vi "test- async-resp for csm loop.vi"(8 "error in (no error)":errorcluster, 11 "TestCase in":refnum<class "testcase-csm loop support.lvclass">) -> (0 "error out":errorcluster, 3 "TestCase out":refnum<class "testcase-csm loop support.lvclass">)   [LabVIEW 2017, in "testcase-csm loop support.lvclass"]
uses:
  testcase-csm loop support.lvclass
  56d4bdba-c2f1-4b55-add1-7a078de9da03.vi
  ea54eaf7-6c78-4206-8259-080cdfbb85de.vi
  src/user.lib/_NEVSTOP/Communicable State Machine(CSM)/AdvanceAPI/CSM - Revert Arguments-Safe String.vi
  src/user.lib/_NEVSTOP/Communicable State Machine(CSM)/_Shared/Trim Single-line Text.vi
  src/user.lib/_NEVSTOP/Communicable State Machine(CSM)/AdvanceAPI/CSM - Make String Arguments Safe.vi
  src/user.lib/_NEVSTOP/Communicable State Machine(CSM)/AdvanceAPI/CSM - Break Down Multiple States String.vi
  src/user.lib/_NEVSTOP/Communicable State Machine(CSM)/AdvanceAPI/CSM - Compact Multiple States.vi
  src/user.lib/_NEVSTOP/Communicable State Machine(CSM)/AdvanceAPI/CSM - Keywords.vi
  <vilib>/addons/_JKI Toolkits/VI Tester/TestCase.llb/TestCase.lvclass
  src/user.lib/_NEVSTOP/Communicable State Machine(CSM)/Communicable State Machine.lvlib
  src/user.lib/_NEVSTOP/Communicable State Machine(CSM)/addons/Loop-Support/CSM Loop Support.lvlib
  C:/Program Files (x86)/National Instruments/LabVIEW 2017/vi.lib/addons/_JKI Toolkits/VI Tester/TestCase.llb/TestCase.lvclass
panel:
  out "Arguments":string
  out "State History 2":string
  out "State History":string
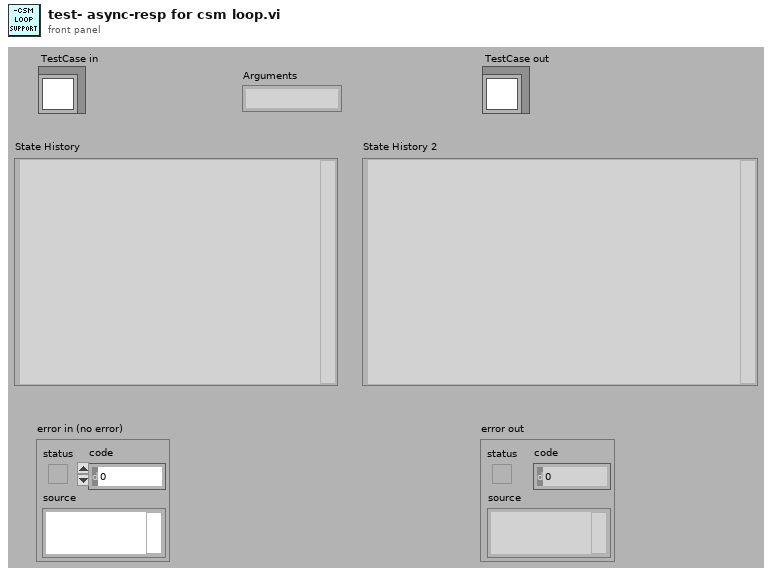
[diagram p1: front panel]
types:
  T1 = enum32{"Invalid", "Standard", "Closed", "Hidden", "Minimized", "Maximized"}
  T2 = enum32{"invalid app kind", "Development System", "Run Time System", "Student Edition", "Embedded LabVIEW", "Evaluation", "Custom"}
  T3 = typedef "Communicable State Machine.lvlib/_CSM_Response Source Message.ctl" = cluster{"‘State":string, "’Arguments":string, "’Error":errorcluster}
  T4 = cluster{"Current VI Reference":refnum<vi>, "Close Panel on Exit?":bool}
  T5 = cluster{"Core":cluster{"Current VI Reference":refnum<vi>, "Close Panel on Exit?":bool}, "diff":dbl, "time":timestamp}
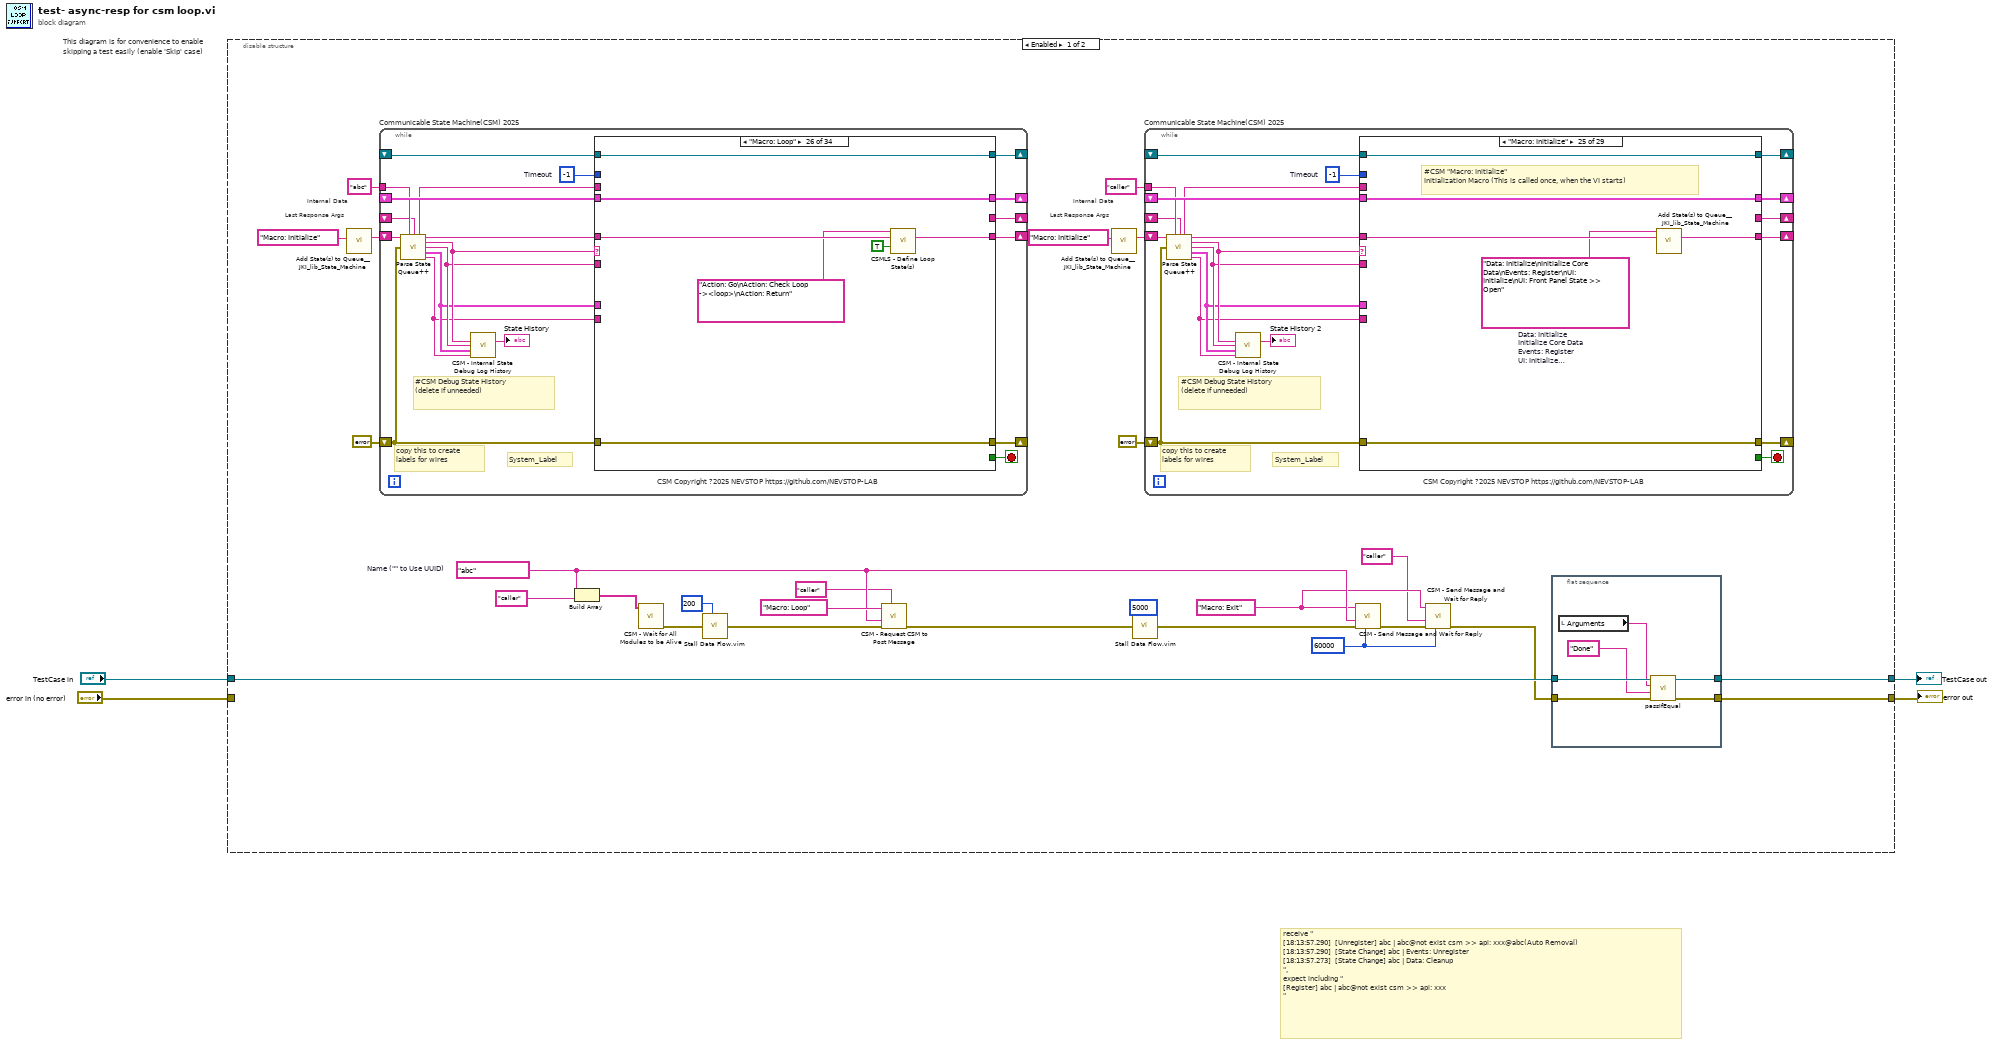
[diagram p0: block diagram]
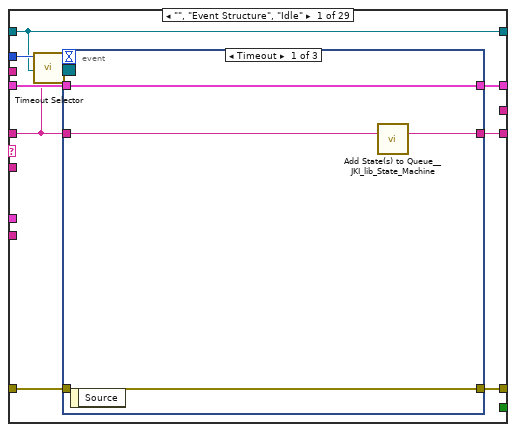
[diagram p2: hidden frame]
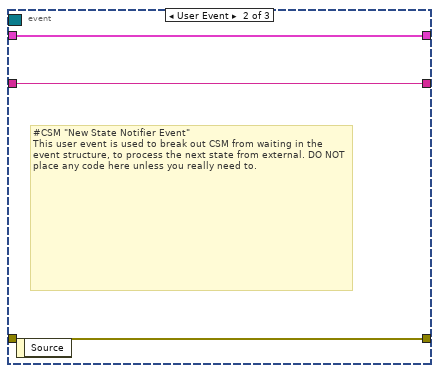
[diagram p3: hidden frame]
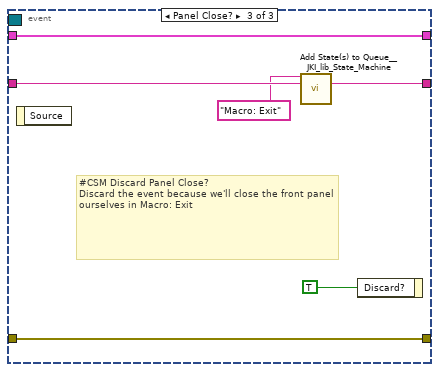
[diagram p4: hidden frame]
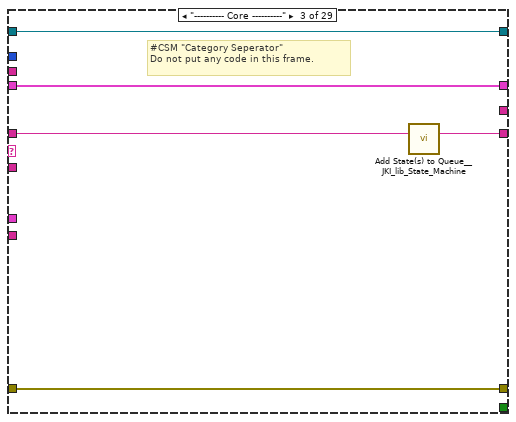
[diagram p6: hidden frame]
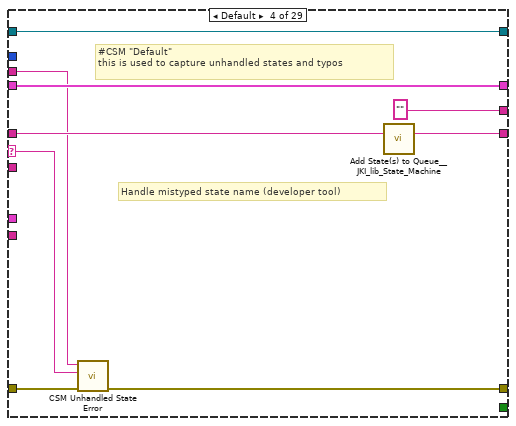
[diagram p7: hidden frame]
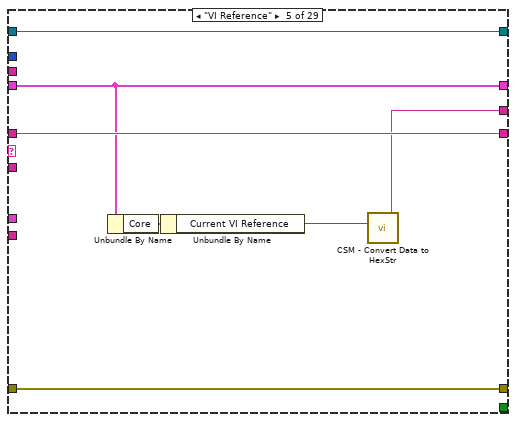
[diagram p8: hidden frame]
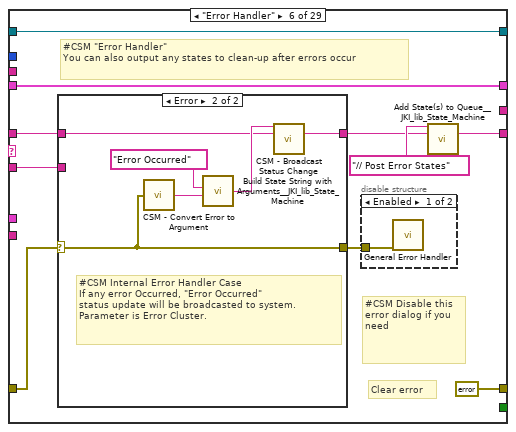
[diagram p9: hidden frame]
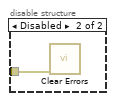
[diagram p10: hidden frame]
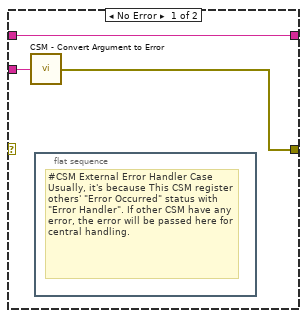
[diagram p11: hidden frame]
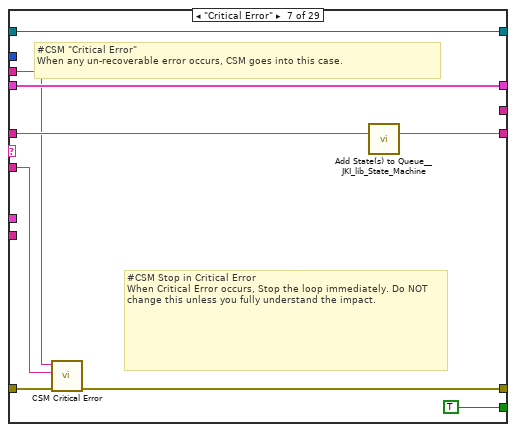
[diagram p12: hidden frame]
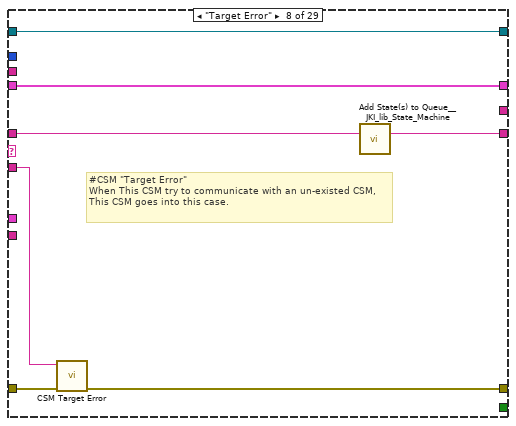
[diagram p13: hidden frame]
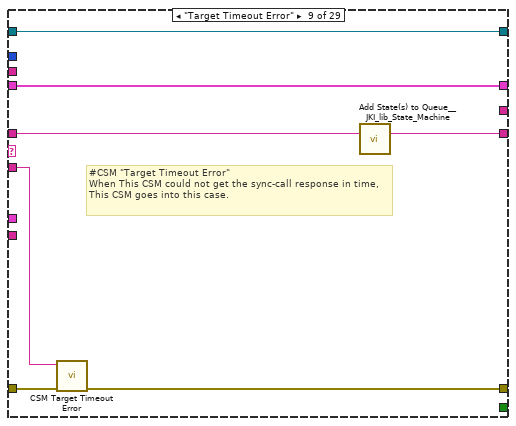
[diagram p14: hidden frame]
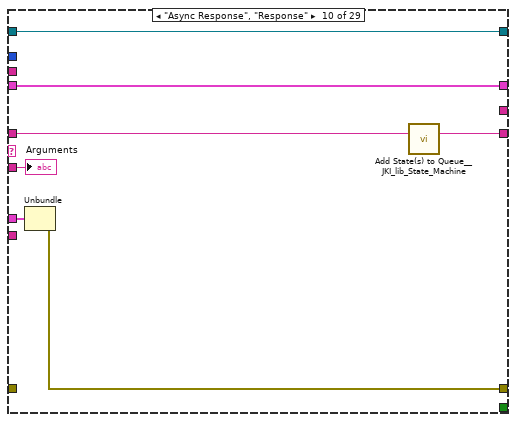
[diagram p15: hidden frame]
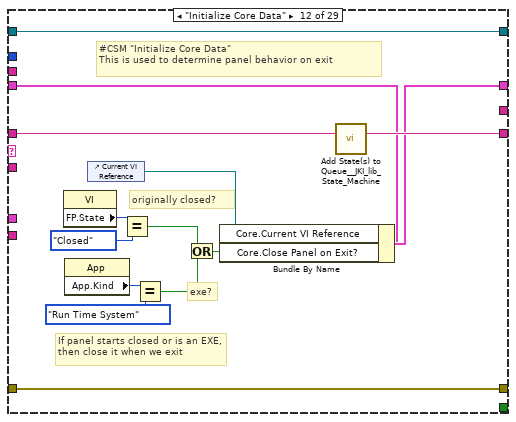
[diagram p17: hidden frame]
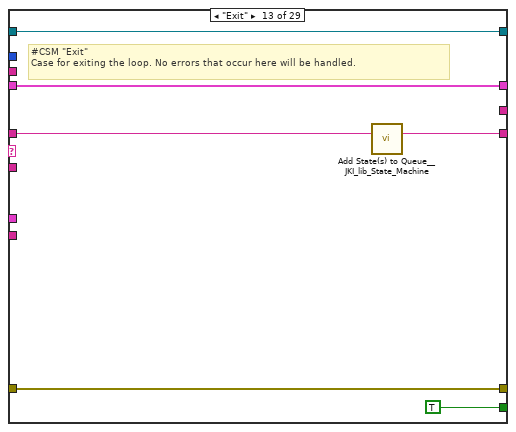
[diagram p18: hidden frame]
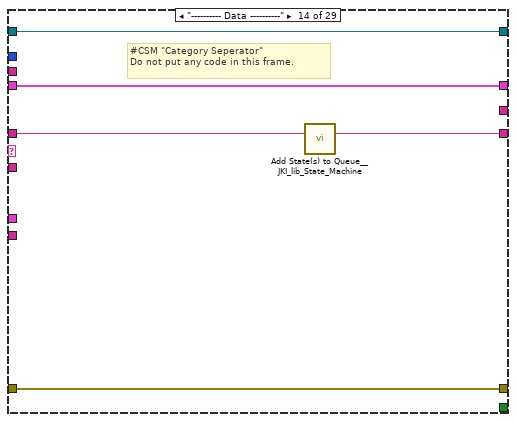
[diagram p19: hidden frame]
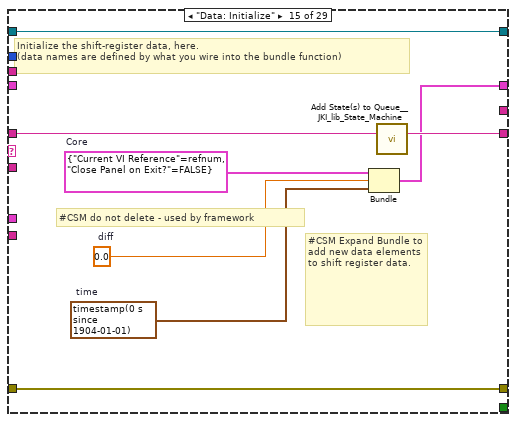
[diagram p20: hidden frame]
diagram:
  # "receive \"\n[18:13:57.290]  [Unregister] abc | abc@not exist csm >> api: xxx@abc(Auto Removal)\n[18:13:57.290]  [State Change] abc | Events: Unregister\n[18:13:57.273]  [State Change] abc | Data: Cleanup\n\", \nexpect including \"\n[Register] abc | abc@not exist csm >> api: xxx\n\""
  n1 = disable-structure "This diagram is for convenience to enable skipping a test easily (enable 'Skip' case)" shown="Enabled" {
    disable-tunnel: "TestCase in" -> [w24 w727]
    disable-tunnel: [w23 w725] -> w1
    disable-tunnel: [w22 w726] -> w3
    disable-tunnel: "error in (no error)" -> [_ w724]
    frame Enabled {
      w5 = 60000 ("Response Timeout (-2 Using Global Settings)")
      w8 = "Macro: Exit" ("State")
      w11 = "abc"  # Name ("" to Use UUID)
      # "Last Response Args"
      # "Internal Data"
      # "Last Response Args"
      # "Internal Data"
      n2 = call <vilib>:"Add State(s) to Queue__JKI_lib_State_Machine.vi"("State(s) in (\"\")"="Macro: Initialize" ("Init State(\"Macro: Initialize\")")) -> ("States Out"=w30:string)  [unwired: 14 in]
      n3 = while "Communicable State Machine(CSM) 2025" {
        shift-right: [w370] -> _
        shift-left: _ -> [w369]
        shift-right: [w373] -> _
        shift-left: errorcluster {"status"=FALSE, "code"=0, "source"=""} ("error out") -> [w367]
        shift-right: [w372] -> _
        shift-left: w30 -> [w374]
        tunnel: "abc" ("Name (\"\" to Use UUID)") -> [w363]
        shift-right: [w366] -> _
        shift-left: _ -> [w357]
        shift-right: [w365] -> _
        shift-left: _ -> [w364]
        stop <- w371 stop-if-true
        w368 = -1  # Timeout
        # "#CSM Debug State History\n(delete if unneeded)"
        # "copy this to create labels for wires"
        # "System_Label"
        # "CSM Copyright ?2025 NEVSTOP https://github.com/NEVSTOP-LAB"
        n4 = call "Parse State Queue++.vi"("State Queue"=w374, "Name (\"\" to Use UUID)"=w363, "Response Arguments"=w357, "Previous Error"=w367) -> ("Name Used"=w358:string, "Remaining States"=w375:string, "Current State"=w362:string, "Arguments"=w361:string, "Additional Information"=w360:T3, "Source CSM"=w359:string)  [unwired: 6 in]
        n5 = call "CSM - Internal State Debug Log History.vi"("State"=w362, "Arguments (\"\")"=w361, ">> Response Source Message >>"=w360, "Source (\"\")"=w359) -> ("Debug Log"=→"State History":string)  [unwired: 11 in]
        n6 = case shown="\"Macro: Loop\"" w362 {
          selector: w362 -> [_ _ _ w409 _ _ _ _ _ _ _ _ _ _ _ _ _ _ _ _ _ _ _ _ _ _ _ _ _ _ _ _ w709 _]
          tunnel: w375 -> [w376 w400 w406 w414 w421 w427 w450 w456 w463 w472 w485 w500 w506 w511 w519 w526 w531 w538 w542 w548 w553 w560 w576 w646 w652 w659 w671 w674 w679 w685 w693 w700 w710 w722]
          tunnel: w361 -> [_ _ _ _ _ w426 w445 w455 w462 w471 _ _ _ _ _ _ _ _ _ _ _ w555 w570 _ _ _ _ _ _ w682 _ _ _ _]
          tunnel: w369 -> [w383 w399 w403 w412 w420 w431 w451 w458 w465 w474 w484 w493 w504 w508 _ w521 w528 w537 w541 w545 w551 w558 w572 w643 w649 w656 w668 w673 w678 w684 w690 w697 w706 w720]
          tunnel: [w382 w401 w404 w407 w422 errorcluster {"status"=FALSE, "code"=0, "source"=""} ("error out") w446 w453 w460 w477 w486 w497 w503 w509 w516 w522 w529 w532 w540 w546 w550 w556 w573 w644 w650 w657 w669 w675 w680 w686 w691 w698 w712 w723] -> w373
          tunnel: w367 -> [w381 w401 w404 w415 w422 w428 w452 w454 w461 _ w486 w497 w503 w509 w516 w523 w529 _ w543 w546 w550 w557 w574 w644 w650 w657 w669 w675 w680 w686 w691 w698 w712 w723]
          tunnel: [w384 w400 w405 w413 w421 w423 w449 w459 w466 w473 w485 w499 w505 w510 w518 w525 w530 w538 w542 w547 w552 w559 w575 w645 w651 w658 w670 w674 w679 w685 w692 w699 w713 w722] -> w372
          tunnel: [_ _ _ _ _ _ TRUE _ _ _ _ _ TRUE _ _ _ _ _ _ _ _ _ _ _ _ _ _ _ _ _ _ _ _ _] -> w371
          tunnel: [w380 w399 w403 w412 w420 w431 w451 w458 w465 w475 w484 w498 w504 w508 w517 w521 w528 w537 w541 w545 w551 w558 w572 w643 w649 w656 w668 w673 w678 w684 w690 w695 w702 w720] -> w370
          tunnel: w368 -> [w379 _ _ _ _ _ _ _ _ _ _ _ _ _ _ _ _ _ _ _ _ _ _ _ _ _ _ _ _ _ _ _ _ _]
          tunnel: w359 -> [_ _ _ _ _ _ _ _ _ w469 _ _ _ _ _ _ _ _ _ _ _ _ _ _ _ _ _ _ _ _ _ _ _ _]
          tunnel: w360 -> [_ _ _ _ _ _ _ _ _ w476 _ _ _ _ _ _ _ _ _ _ _ _ _ _ _ _ _ _ _ _ _ _ _ _]
          tunnel: [_ _ _ "" w416 _ _ _ _ _ _ _ _ _ _ _ _ _ _ _ _ _ _ _ _ _ _ _ "API1 Response" w681 _ _ _ "Done" ("HEX String (0-9,A-F)")] -> w366
          tunnel: [w378 w398 w402 w410 w419 w430 w447 w457 w464 w478 w483 w487 w501 w507 w512 w520 w527 w536 w539 w544 w549 w554 w569 w642 w647 w654 w661 w672 w677 w683 w689 w696 w711 w721] -> w365
          tunnel: w364 -> [w378 w398 w402 w410 w419 w430 w447 w457 w464 w478 w483 w487 w501 w507 w512 w520 w527 _ w539 w544 w549 w554 w569 w642 w647 w654 w661 w672 w677 w683 w689 w696 w711 w721]
          tunnel: w358 -> [_ _ _ w408 _ _ w444 _ _ _ _ _ _ _ _ _ _ w535 _ _ _ _ _ _ _ _ _ _ _ _ _ _ _ _]
          frame "", "Event Structure", "Idle" {
            n7 = call "Timeout Selector.vi"("Remaining States"=w376, "Timeout Expected"=w379) -> ("Timeout"=w377:i32)  [unwired: 5 in]
            n8 = event shown="[1] <New State Notifier Event>: User Event" {
              selector: w378 -> [_ _ _]
              dyn-events: _ -> [_ _ _]
              timeout: w377 -> [_ _ _]
              tunnel: w376 -> [w388 w390 w397]
              tunnel: [w387 w390 w396] -> w384
              tunnel: w383 -> [w385 w391 w394]
              tunnel: [w386 w389 w395] -> w382
              tunnel: w381 -> [w386 w389 w395]
              tunnel: [w385 w391 w394] -> w380
              event Timeout {
                n9 = event-data() -> ()  [unwired: 1 in, 1 out]
                n10 = call <vilib>:"Add State(s) to Queue__JKI_lib_State_Machine.vi"("State(s) in (\"\")"=w388) -> ("States Out"=w387:string)  [unwired: 14 in]
              }
              event User Event {
                # "#CSM \"New State Notifier Event\"\nThis user event is used to break out CSM from waiting in the event structure, to process the next state from external. DO NOT place any code here unless you really need to."
                n11 = event-data() -> ()  [unwired: 1 in, 1 out]
              }
              event Panel Close? {
                # "#CSM Discard Panel Close?\nDiscard the event because we'll close the front panel ourselves in Macro: Exit"
                n12 = event-data() -> ()  [unwired: 1 in, 1 out]
                n13 = call <vilib>:"Add State(s) to Queue__JKI_lib_State_Machine.vi"("State(s) in Front (\"\")"="Macro: Exit", "State(s) in (\"\")"=w397) -> ("States Out"=w396:string)  [unwired: 13 in]
                n14 = event-data("Discard?"=TRUE) -> ()  [unwired: 1 in, 1 out]
              }
            }
          }
          frame "CSM Documentation" {
            # "#CSM README FIRST\n\nCommunicable State Machine(CSM) is a LabVIEW application framework that builds upon JKI State Machine(JKISM). It follows the pattern of JKISM and extends the keywords to describe message communication between modules, including concepts such as Sync-Message, Async-Message, Subscription/Unsubscription of status - essential elements for creating reusable code modules. For more information, please visit the CSM wiki: https://nevstop-lab.github.io/CSM-Wiki/\n\nFor instructions on JKI State Machine, visit: http://jki.net/state-machine/\nFor information about CSM, visit: https://github.com/NEVSTOP-LAB"
            # "#CSM \"Documentation\"\nCase for holding CSM Documenation"
          }
          frame "---------- Core ----------" {
            # "#CSM \"Category Seperator\"\nDo not put any code in this frame."
            n15 = call <vilib>:"Add State(s) to Queue__JKI_lib_State_Machine.vi"("State(s) in (\"\")"=w406) -> ("States Out"=w405:string)  [unwired: 14 in]
          }
          frame Default {
            # "#CSM \"Default\"\nthis is used to capture unhandled states and typos"
            # "Handle mistyped state name (developer tool)"
            n16 = call "CSM Unhandled State Error.vi"("error in (no error)"=w415, "Undefined State"=w409, "CSM Name"=w408) -> ("error out"=w407:errorcluster)  [unwired: 8 in]
            n17 = call <vilib>:"Add State(s) to Queue__JKI_lib_State_Machine.vi"("State(s) in (\"\")"=w414) -> ("States Out"=w413:string)  [unwired: 14 in]
          }
          frame "VI Reference" {
            n18 = Unbundle By Name(w420) -> ("Core"=w418:T4)
            n19 = Unbundle By Name(w418) -> ("Current VI Reference"=w417:refnum<vi>)
            n20 = call "CSM - Convert Data to HexStr.vi"("Variant"=w417) -> ("HEX String (0-9,A-F)"=w416:string)  [unwired: 8 in]
          }
          frame "Error Handler" {
            # "#CSM Disable this error dialog if you need"
            # "#CSM \"Error Handler\"\nYou can also output any states to clean-up after errors occur"
            # "Clear error"
            n21 = case shown="Error" w428 {
              selector: w428 -> [_ w438]
              tunnel: [w437 w440] -> w424
              tunnel: w427 -> [w437 w439]
              tunnel: w426 -> [w436 _]
              tunnel: [w435 w438] -> w429
              frame No Error {
                n22 = call "CSM - Convert Argument to Error.vi"("Argument"=w436) -> ("Error"=w435:errorcluster)  [unwired: 4 in]
                n23 = flat-sequence {
                  frame #0 {
                    # "#CSM External Error Handler Case\nUsually, it's because This CSM register others' \"Error Occurred\" status with \"Error Handler\". If other CSM have any error, the error will be passed here for central handling."
                  }
                }
              }
              frame Error {
                # "#CSM Internal Error Handler Case \nIf any error Occurred, \"Error Occurred\" \nstatus update will be broadcasted to system.\nParameter is Error Cluster."
                n24 = call "CSM - Convert Error to Argument.vi"("Error"=w438) -> ("Argument"=w442:string)  [unwired: 4 in]
                n25 = call <vilib>:"Build State String with Arguments__JKI_lib_State_Machine.vi"("Arguments (\"\")"=w442, "State"="Error Occurred" ("Status with Arguments")) -> ("State with Arguments"=w441:string)  [unwired: 4 in]
                n26 = call "CSM - Broadcast Status Change.vi"("Status With Arguments"=w441, "State Queue"=w439) -> ("Remaining States"=w440:string)  [unwired: 13 in]
              }
            }
            n27 = disable-structure shown="Enabled" {
              disable-tunnel: w429 -> [w433 w434]
              frame Enabled {
                n28 = call <vilib>:"General Error Handler.vi"("error in (no error)"=w433) -> ()  [unwired: 10 in, 5 out]
              }
              frame Disabled {
                n29 = call <vilib>:"Clear Errors.vi"("error in (no error)"=w434) -> ()  [unwired: 5 in, 2 out]
              }
            }
            n30 = call <vilib>:"Add State(s) to Queue__JKI_lib_State_Machine.vi"("State(s) in Front (\"\")"="// Post Error States", "State(s) in (\"\")"=w424) -> ("States Out"=w423:string)  [unwired: 13 in]
          }
          frame "Critical Error" {
            # "#CSM Stop in Critical Error\nWhen Critical Error occurs, Stop the loop immediately. Do NOT change this unless you fully understand the impact."
            # "#CSM \"Critical Error\"\nWhen any un-recoverable error occurs, CSM goes into this case."
            n31 = call "CSM Critical Error.vi"("error in (no error)"=w452, "Arugments (As Reason)"=w445, "CSM Name"=w444) -> ("error out"=w446:errorcluster)  [unwired: 8 in]
            n32 = call <vilib>:"Add State(s) to Queue__JKI_lib_State_Machine.vi"("State(s) in (\"\")"=w450) -> ("States Out"=w449:string)  [unwired: 14 in]
          }
          frame "Target Error" {
            # "#CSM \"Target Error\"\nWhen This CSM try to communicate with an un-existed CSM, This CSM goes into this case."
            n33 = call "CSM Target Error.vi"("error in (no error)"=w454, "Arguments (As CSM Name)"=w455) -> ("error out"=w453:errorcluster)  [unwired: 9 in]
            n34 = call <vilib>:"Add State(s) to Queue__JKI_lib_State_Machine.vi"("State(s) in (\"\")"=w456) -> ("States Out"=w459:string)  [unwired: 14 in]
          }
          frame "Target Timeout Error" {
            # "#CSM \"Target Timeout Error\"\nWhen This CSM could not get the sync-call response in time, This CSM goes into this case."
            n35 = call "CSM Target Timeout Error.vi"("error in (no error)"=w461, "Arguments (As CSM Name)"=w462) -> ("error out"=w460:errorcluster)  [unwired: 9 in]
            n36 = call <vilib>:"Add State(s) to Queue__JKI_lib_State_Machine.vi"("State(s) in (\"\")"=w463) -> ("States Out"=w466:string)  [unwired: 14 in]
          }
          frame "Async Response", "Response" {
            n37 = Unbundle(w476) -> ("‘State"=w470:string, "’Arguments"=w468:string, "’Error"=w467:errorcluster)
            n38 = case shown="Default" w470 {
              tunnel: [w482] -> w477
              tunnel: w467 -> [w482]
              tunnel: [w481] -> w475
              tunnel: w474 -> [w481]
              tunnel: [w479] -> w473
              tunnel: w472 -> [w480]
              tunnel: w471 -> [_]
              tunnel: w469 -> [_]
              tunnel: w468 -> [_]
              frame Default {
                # "#CSM Response Comments\nAfter Message is executed, CSM goes to this state for receive the response.\n    For Async Message(->), \"Async Response\" is used. This CSM will goes to \"Async Message Posted\" immediately and receive the \"Async Response\" after the callee finishes the message.\n    For Sync Message(@),  This CSM will wait until the message is done and immediately goes to \"Response\""
                # "#CSM \"Async Response\"\nHandle Async-call Response (\"Async Response\" for ->)"
                # "#CSM \"Response\"\nHandle Sync-call Response (\"Response\" for -@)"
                n39 = call <vilib>:"Add State(s) to Queue__JKI_lib_State_Machine.vi"("State(s) in (\"\")"=w480) -> ("States Out"=w479:string)  [unwired: 14 in]
              }
            }
          }
          frame "Async Message Posted" {
            # "#CSM \"Async Message Posted\"\nAfter Async Message is posted (-> or ->| ), CSM goes to this state for post-action.\nYou can use Argument - State to tell which Async Message is called."
          }
          frame "Initialize Core Data" {
            # "#CSM \"Initialize Core Data\"\nThis is used to determine panel behavior on exit"
            # "originally closed?"
            # "exe?"
            # "If panel starts closed or is an EXE, then close it when we exit"
            n40 = property class="VI"() -> ("FP.State"=w490:T1)  [unwired: 2 in, 2 out]
            n41 = property class="App"() -> ("App.Kind"=w496:T2)  [unwired: 2 in, 2 out]
            n42 = control-ref of="Current VI Reference"() -> (w491:refnum<vi>)
            n43 = Equal?(x=w490, y=T1."Closed" ("Front Panel Window:State")) -> (x = y?=w488:bool)
            n44 = Equal?(x=w496, y=T2."Run Time System" ("Application:Kind")) -> (x = y?=w494:bool)
            n45 = Or(x=w488, y=w494) -> (x .or. y?=w492:bool)
            n46 = Bundle By Name(cluster=w493, "Core.Current VI Reference"=w491, "Core.Close Panel on Exit?"=w492) -> (w498:T5)
            n47 = call <vilib>:"Add State(s) to Queue__JKI_lib_State_Machine.vi"("State(s) in (\"\")"=w500) -> ("States Out"=w499:string)  [unwired: 14 in]
          }
          frame "Exit" {
            # "#CSM \"Exit\"\nCase for exiting the loop. No errors that occur here will be handled."
            n48 = call <vilib>:"Add State(s) to Queue__JKI_lib_State_Machine.vi"("State(s) in (\"\")"=w506) -> ("States Out"=w505:string)  [unwired: 14 in]
          }
          frame "---------- Data ----------" {
            # "#CSM \"Category Seperator\"\nDo not put any code in this frame."
            n49 = call <vilib>:"Add State(s) to Queue__JKI_lib_State_Machine.vi"("State(s) in (\"\")"=w511) -> ("States Out"=w510:string)  [unwired: 14 in]
          }
          frame "Data: Initialize" {
            w513 = T4 {"Current VI Reference"=refnum, "Close Panel on Exit?"=FALSE}  # Core
            w515 = 0.0  # diff
            w514 = timestamp(0 s since 1904-01-01)  # time
            # "#CSM do not delete - used by framework"
            # "#CSM Expand Bundle to add new data elements to shift register data."
            # "Initialize the shift-register data, here.\n(data names are defined by what you wire into the bundle function)"
            n50 = Bundle("Core"=w513, "diff"=w515, "time"=w514) -> (w517:T5)  [unwired: 1 in]
            n51 = call <vilib>:"Add State(s) to Queue__JKI_lib_State_Machine.vi"("State(s) in (\"\")"=w519) -> ("States Out"=w518:string)  [unwired: 14 in]
          }
          frame "Data: Cleanup" {
            # "Cleanup any data and references, here.\n(this is called automatically, by the Macro: Exit)"
            n52 = Unbundle By Name(w521) -> ("Core.Current VI Reference"=w524:refnum<vi>)
            n53 = Close Reference(reference=w524, error in (no error)=w523) -> (error out=w522:errorcluster)
            n54 = call <vilib>:"Add State(s) to Queue__JKI_lib_State_Machine.vi"("State(s) in (\"\")"=w526) -> ("States Out"=w525:string)  [unwired: 14 in]
          }
          frame "---------- Events ----------" {
            # "#CSM \"Category Seperator\"\nDo not put any code in this frame."
            n55 = call <vilib>:"Add State(s) to Queue__JKI_lib_State_Machine.vi"("State(s) in (\"\")"=w531) -> ("States Out"=w530:string)  [unwired: 14 in]
          }
          frame "Events: Register" {
            # "#CSM \"Events: Register\"\nRegister user event. New Message Event is registered to break CSM waiting in event structure by default."
            # "#CSM Register New Message Event\nRegister message event to break Waiting in Event structure."
            n56 = call "CSM - Get New State Notifier Event.vi"("Name (\"\" to Use UUID)"=w535) -> ("error out"=w533:errorcluster, "New State Notifier Event"=w534:refnum<user-event>)  [unwired: 9 in]
            n57 = register-events(error in=w533, w534) -> (reference out=w536:refnum<event-registration>, error out=w532:errorcluster)  [unwired: 1 in]
          }
          frame "Events: Unregister" {
            # "#CSM \"Events: Unregister\"\nUnregister user event."
            n58 = Unregister For Events(event registration refnum=w539, error in=w543) -> (error out=w540:errorcluster)
          }
          frame "---------- UI ----------" {
            # "#CSM \"Category Seperator\"\nDo not put any code in this frame."
            n59 = call <vilib>:"Add State(s) to Queue__JKI_lib_State_Machine.vi"("State(s) in (\"\")"=w548) -> ("States Out"=w547:string)  [unwired: 14 in]
          }
          frame "UI: Initialize" {
            # "#CSM \"UI: Initialize\"\nInitialize the User Interface, here.\n(this is called automatically, by the Macro: Init)"
            n60 = call <vilib>:"Add State(s) to Queue__JKI_lib_State_Machine.vi"("State(s) in (\"\")"=w553) -> ("States Out"=w552:string)  [unwired: 14 in]
          }
          frame "UI: Cursor Set" {
            # "#CSM \"UI: Cursor Set\"\nSet and Unset Cursor Busy.\n(Usage: \"UI: Cursor Set >> Busy|Idle\")"
            # "Argument"
            n61 = disable-structure shown="Default" {
              disable-tunnel: w557 -> [w563 w568]
              disable-tunnel: [w562 w568] -> w556
              disable-tunnel: w555 -> [w561 _]
              frame condition #0 (active) {
                n62 = case shown="\"Idle\", Default" w561 {
                  tunnel: w563 -> [w565 w567]
                  tunnel: [w564 w566] -> w562
                  frame "Idle", Default {
                    n63 = call <vilib>:"Unset Busy.vi"("error in (no error)"=w565) -> ("error out"=w564:errorcluster)  [unwired: 10 in]
                  }
                  frame "Busy" {
                    n64 = call <vilib>:"Set Busy.vi"("error in (no error)"=w567) -> ("error out"=w566:errorcluster)  [unwired: 9 in, 1 out]
                  }
                }
              }
              frame condition #1 {
              }
            }
            n65 = call <vilib>:"Add State(s) to Queue__JKI_lib_State_Machine.vi"("State(s) in (\"\")"=w560) -> ("States Out"=w559:string)  [unwired: 14 in]
          }
          frame "UI: Front Panel State" {
            # "#CSM \"UI: Front Panel State\"\nSet Front Panel Open or Closed\n(Usage: \"UI: Front Panel State >> Open|Close\")"
            # "Argument"
            n66 = Unbundle By Name(w572) -> ("Core.Current VI Reference"=w571:refnum<vi>)
            n67 = call <vilib>:"Add State(s) to Queue__JKI_lib_State_Machine.vi"("State(s) in (\"\")"=w576) -> ("States Out"=w575:string)  [unwired: 14 in]
            n68 = case shown="\"Close\", \"Closed\"" w570 {
              tunnel: w574 -> [w582 w597 w608 w621 w634]
              tunnel: [w584 w598 w610 w623 w636] -> w573
              tunnel: w571 -> [w583 w595 w609 w622 w635]
              frame "Open", "Standard", Default {
                w577 = T1."Standard" ("State")
                n69 = property class="VI"(reference=w583, error in=w582) -> (reference out=w580:refnum<vi>, error out=w581:errorcluster, "FP.State"=w579:T1)
                n70 = Not Equal?(x=w579, y=w577) -> (x != y?=w578:bool)
                n71 = case shown="True" w578 {
                  tunnel: [w588 w590] -> w584
                  tunnel: w581 -> [w587 w590]
                  tunnel: w580 -> [w586 _]
                  tunnel: w577 -> [w585 _]
                  frame True {
                    n72 = invoke class="VI" method="FP.Open"(reference=w586, error in=w587, "Activate"=TRUE, "State"=w585) -> (error out=w588:errorcluster)  [unwired: 1 in, 4 out]
                  }
                  frame False {
                  }
                }
              }
              frame "Close", "Closed" {
                n73 = property class="VI"(reference=w595, error in=w597) -> (reference out=w594:refnum<vi>, error out=w596:errorcluster, "FP.State"=w592:T1)
                n74 = Not Equal?(x=w592, y=T1."Closed" ("Front Panel Window:State")) -> (x != y?=w591:bool)
                n75 = case shown="False" w591 {
                  tunnel: [w599 w602] -> w598
                  tunnel: w596 -> [w599 w601]
                  tunnel: w594 -> [_ w600]
                  frame False {
                  }
                  frame True {
                    n76 = invoke class="VI" method="FP.Close"(reference=w600, error in=w601) -> (error out=w602:errorcluster)  [unwired: 1 in, 2 out]
                  }
                }
              }
              frame "Hidden", "Hide" {
                w603 = T1."Hidden" ("State")
                n77 = property class="VI"(reference=w609, error in=w608) -> (reference out=w606:refnum<vi>, error out=w607:errorcluster, "FP.State"=w605:T1)
                n78 = Not Equal?(x=w605, y=w603) -> (x != y?=w604:bool)
                n79 = case shown="True" w604 {
                  tunnel: [w614 w615] -> w610
                  tunnel: w607 -> [w613 w615]
                  tunnel: w606 -> [w612 _]
                  tunnel: w603 -> [w611 _]
                  frame True {
                    n80 = invoke class="VI" method="FP.Open"(reference=w612, error in=w613, "State"=w611) -> (error out=w614:errorcluster)  [unwired: 2 in, 4 out]
                  }
                  frame False {
                  }
                }
              }
              frame "Minimize", "Minimized" {
                w616 = T1."Minimized" ("State")
                n81 = property class="VI"(reference=w622, error in=w621) -> (reference out=w619:refnum<vi>, error out=w620:errorcluster, "FP.State"=w618:T1)
                n82 = Not Equal?(x=w618, y=w616) -> (x != y?=w617:bool)
                n83 = case shown="True" w617 {
                  tunnel: [w627 w628] -> w623
                  tunnel: w620 -> [w626 w628]
                  tunnel: w619 -> [w625 _]
                  tunnel: w616 -> [w624 _]
                  frame True {
                    n84 = invoke class="VI" method="FP.Open"(reference=w625, error in=w626, "State"=w624) -> (error out=w627:errorcluster)  [unwired: 2 in, 4 out]
                  }
                  frame False {
                  }
                }
              }
              frame "Maximize", "Maximized" {
                w629 = T1."Maximized" ("State")
                n85 = property class="VI"(reference=w635, error in=w634) -> (reference out=w632:refnum<vi>, error out=w633:errorcluster, "FP.State"=w631:T1)
                n86 = Not Equal?(x=w631, y=w629) -> (x != y?=w630:bool)
                n87 = case shown="True" w630 {
                  tunnel: [w640 w641] -> w636
                  tunnel: w633 -> [w639 w641]
                  tunnel: w632 -> [w638 _]
                  tunnel: w629 -> [w637 _]
                  frame True {
                    n88 = invoke class="VI" method="FP.Open"(reference=w638, error in=w639, "State"=w637) -> (error out=w640:errorcluster)  [unwired: 2 in, 4 out]
                  }
                  frame False {
                  }
                }
              }
            }
          }
          frame "---------- Macro ----------" {
            # "#CSM \"Category Seperator\"\nDo not put any code in this frame."
            n89 = call <vilib>:"Add State(s) to Queue__JKI_lib_State_Machine.vi"("State(s) in (\"\")"=w646) -> ("States Out"=w645:string)  [unwired: 14 in]
          }
          frame "Macro: Initialize" {
            w648 = "Data: Initialize\nInitialize Core Data\nEvents: Register\nUI: Initialize\nUI: Front Panel State >> Open"  # Data: Initialize Initialize Core Data Events: Register UI: Initialize UI: Front Panel State >> Open
            # "#CSM \"Macro: Initialize\"\nInitialization Macro (This is called once, when the VI starts)"
            n90 = call <vilib>:"Add State(s) to Queue__JKI_lib_State_Machine.vi"("State(s) in Front (\"\")"=w648, "State(s) in (\"\")"=w652) -> ("States Out"=w651:string)  [unwired: 13 in]
          }
          frame "Macro: Loop" {
            n91 = call "CSMLS - Define Loop State(s).vi"("Loop States"="Action: Go\nAction: Check Loop -><loop>\nAction: Return", "States Queue"=w659, "Add to Front? (F)"=TRUE ("Front(T)/Back(F)")) -> ("Remaining States"=w658:string)  [unwired: 12 in]
          }
          frame "Macro: Exit" {
            # "#CSM \"Macro: Exit\"\nExit Macro (This is called once, when the VI exits)"
            n92 = Unbundle By Name(w668) -> ("Core.Close Panel on Exit?"=w667:bool)
            n93 = Select(t="UI: Front Panel State >> Close", s=w667, f="") -> (s? t:f=w664:string)
            n94 = call <vilib>:"Add State(s) to Queue__JKI_lib_State_Machine.vi"("State(s) in Front (\"\")"="//Exit Sub-Modules ", "State(s) in (\"\")"=w664, "State(s) at Back (\"\")"="Data: Cleanup\nEvents: Unregister\nExit") -> ("States Out"=w662:string)  [unwired: 12 in]
            n95 = call <vilib>:"Add State(s) to Queue__JKI_lib_State_Machine.vi"("State(s) in Front (\"\")"=w662, "State(s) in (\"\")"=w671) -> ("States Out"=w670:string)  [unwired: 13 in]
          }
          frame "---------- API ----------" {
            # "#CSM \"Category Seperator\"\nDo not put any code in this frame."
          }
          frame "API: API1" {
            # "#CSM API Example\nCopy/Rename this case for your own API"
            # "#CSM Response\nConnect this to return the response of your API"
            # "#CSM >> Source CSM >>\nIf you need to tell who triggered this state , use this string. If it's this case itself, this string is \"\"."
            # "#CSM >> Arguments >>\nDeal with the parameter if any"
          }
          frame "API: API2" {
            # "#CSM API Example\nCopy/Rename this case for your own API"
            # "unpack Hex String  to Variant\nif complex parameter is needed."
            n96 = call "CSM - Convert HexStr to Data.vi"("HEX String"=w682) -> ()  [unwired: 7 in, 2 out]
            n97 = disable-structure shown="Disabled" {
              disable-tunnel: [w687 "API2 Response"] -> w681
              frame Disabled {
                # "pack variant to hexstr \nif complex response is needed."
                # "complex Response"
                n98 = call "CSM - Convert Data to HexStr.vi"() -> ("HEX String (0-9,A-F)"=w687:string)  [unwired: 9 in]
              }
              frame Enabled {
              }
            }
          }
          frame "---------- Action ----------" {
            # "#CSM \"Category Seperator\"\nDo not put any code in this frame."
            n99 = call <vilib>:"Add State(s) to Queue__JKI_lib_State_Machine.vi"("State(s) in (\"\")"=w693) -> ("States Out"=w692:string)  [unwired: 14 in]
          }
          frame "Action: Go" {
            n100 = Get Date/Time In Seconds() -> (seconds since 1Jan1904=w694:timestamp)
            n101 = Bundle By Name(cluster=w697, "time"=w694) -> (w695:T5)
            n102 = call <vilib>:"Add State(s) to Queue__JKI_lib_State_Machine.vi"("State(s) in (\"\")"=w700) -> ("States Out"=w699:string)  [unwired: 14 in]
          }
          frame "Action: Check Loop" {
            n103 = Unbundle By Name(w706) -> ("time"=w705:timestamp)
            n104 = Wait (ms)(milliseconds to wait=u32 100) -> ()  [unwired: 1 out]
            n105 = Get Date/Time In Seconds() -> (seconds since 1Jan1904=w707:timestamp)
            n106 = Subtract(x=w707, y=w705) -> (x-y=w701:dbl)
            n107 = Greater?(x=w701, y=3.0) -> (0:w703:bool)
            n108 = case shown="False" w703 {
              tunnel: [w717 w718] -> w713
              tunnel: w710 -> [w716 w718]
              tunnel: w709 -> [w714 _]
              frame False {
                n109 = call "CSMLS - Append Continuous State.vi"("Loop State(s) And Arguments"="" ("Loop State(s) and Arguments"), "Continous State"=w714, "States Queue"=w716) -> ("Remaining States"=w717:string)  [unwired: 8 in]
              }
              frame True {
              }
            }
            n110 = Bundle By Name(cluster=w706, "diff"=w701) -> (w702:T5)
          }
          frame "Action: Return" {
          }
        }
      }
      n111 = Build Array(w11, "caller" ("Name (\"\" to Use UUID)")) -> (w13:string[])
      n112 = call "CSM - Wait for All Modules to be Alive.vi"("CSM Names"=w13) -> ("error out"=w26:errorcluster)  [unwired: 8 in, 2 out]
      n113 = call "Stall Data Flow.vim"("value in"=w26, "milliseconds to wait"=u32 200) -> ("value out"=w19:errorcluster)  [unwired: 1 out]
      n114 = call "CSM - Request CSM to Post Message.vi"("Module Name"="caller" ("Name (\"\" to Use UUID)"), "Error In (No Error)"=w19, "Target Module (\"\" By Default)"=w11, "State"="Macro: Loop") -> ("error out"=w25:errorcluster)  [unwired: 7 in]
      n115 = call <vilib>:"Add State(s) to Queue__JKI_lib_State_Machine.vi"("State(s) in (\"\")"="Macro: Initialize" ("Init State(\"Macro: Initialize\")")) -> ("States Out"=w14:string)  [unwired: 14 in]
      n116 = call "Stall Data Flow.vim"("value in"=w25, "milliseconds to wait"=u32 5000) -> ("value out"=w21:errorcluster)  [unwired: 1 out]
      n117 = while "Communicable State Machine(CSM) 2025" {
        shift-right: [w52] -> _
        shift-left: _ -> [w51]
        shift-right: [w55] -> _
        shift-left: errorcluster {"status"=FALSE, "code"=0, "source"=""} ("error out") -> [w49]
        shift-right: [w54] -> _
        shift-left: w14 -> [w56]
        tunnel: "caller" ("Name (\"\" to Use UUID)") -> [w45]
        shift-right: [w48] -> _
        shift-left: _ -> [w39]
        shift-right: [w47] -> _
        shift-left: _ -> [w46]
        stop <- w53 stop-if-true
        w50 = -1  # Timeout
        # "#CSM Debug State History\n(delete if unneeded)"
        # "copy this to create labels for wires"
        # "System_Label"
        # "CSM Copyright ?2025 NEVSTOP https://github.com/NEVSTOP-LAB"
        n118 = call "Parse State Queue++.vi"("State Queue"=w56, "Name (\"\" to Use UUID)"=w45, "Response Arguments"=w39, "Previous Error"=w49) -> ("Name Used"=w40:string, "Remaining States"=w57:string, "Current State"=w44:string, "Arguments"=w43:string, "Additional Information"=w42:T3, "Source CSM"=w41:string)  [unwired: 6 in]
        n119 = call "CSM - Internal State Debug Log History.vi"("State"=w44, "Arguments (\"\")"=w43, ">> Response Source Message >>"=w42, "Source (\"\")"=w41) -> ("Debug Log"=→"State History 2":string)  [unwired: 11 in]
        n120 = case shown="\"Macro: Initialize\"" w44 {
          selector: w44 -> [_ _ _ w91 _ _ _ _ _ _ _ _ _ _ _ _ _ _ _ _ _ _ _ _ _ _ _ _ _]
          tunnel: w57 -> [w58 w82 w88 w96 w103 w109 w132 w138 w145 w151 w158 w173 w179 w184 w192 w199 w204 w211 w215 w221 w227 w234 w250 w320 w326 w338 w341 w346 w352]
          tunnel: w43 -> [_ _ _ _ _ w108 w127 w137 w144 w149 _ _ _ _ _ _ _ _ _ _ _ w229 w244 _ _ _ _ _ w349]
          tunnel: w51 -> [w65 w81 w85 w94 w102 w113 w133 w140 w147 w153 w157 w166 w177 w181 _ w194 w201 w210 w214 w218 w225 w232 w246 w317 w323 w335 w340 w345 w351]
          tunnel: [w64 w83 w86 w89 w104 errorcluster {"status"=FALSE, "code"=0, "source"=""} ("error out") w128 w135 w142 w150 w159 w170 w176 w182 w189 w195 w202 w205 w213 w219 w224 w230 w247 w318 w324 w336 w342 w347 w353] -> w55
          tunnel: w49 -> [w63 w83 w86 w97 w104 w110 w134 w136 w143 _ w159 w170 w176 w182 w189 w196 w202 _ w216 w219 w224 w231 w248 w318 w324 w336 w342 w347 w353]
          tunnel: [w66 w82 w87 w95 w103 w105 w131 w141 w148 w152 w158 w172 w178 w183 w191 w198 w203 w211 w215 w220 w226 w233 w249 w319 w325 w337 w341 w346 w352] -> w54
          tunnel: [_ _ _ _ _ _ TRUE _ _ _ _ _ TRUE _ _ _ _ _ _ _ _ _ _ _ _ _ _ _ _] -> w53
          tunnel: [w62 w81 w85 w94 w102 w113 w133 w140 w147 w153 w157 w171 w177 w181 w190 w194 w201 w210 w214 w218 w225 w232 w246 w317 w323 w335 w340 w345 w351] -> w52
          tunnel: w50 -> [w61 _ _ _ _ _ _ _ _ _ _ _ _ _ _ _ _ _ _ _ _ _ _ _ _ _ _ _ _]
          tunnel: w41 -> [_ _ _ _ _ _ _ _ _ _ _ _ _ _ _ _ _ _ _ _ _ _ _ _ _ _ _ _ _]
          tunnel: w42 -> [_ _ _ _ _ _ _ _ _ w154 _ _ _ _ _ _ _ _ _ _ _ _ _ _ _ _ _ _ _]
          tunnel: [_ _ _ "" w98 _ _ _ _ _ _ _ _ _ _ _ _ _ _ _ _ _ _ _ _ _ _ "API1 Response" w348] -> w48
          tunnel: [w60 w80 w84 w92 w101 w112 w129 w139 w146 w155 w156 w160 w174 w180 w185 w193 w200 w209 w212 w217 w223 w228 w243 w316 w321 w328 w339 w344 w350] -> w47
          tunnel: w46 -> [w60 w80 w84 w92 w101 w112 w129 w139 w146 w155 w156 w160 w174 w180 w185 w193 w200 _ w212 w217 w223 w228 w243 w316 w321 w328 w339 w344 w350]
          tunnel: w40 -> [_ _ _ w90 _ _ w126 _ _ _ _ _ _ _ _ _ _ w208 _ _ _ _ _ _ _ _ _ _ _]
          frame "", "Event Structure", "Idle" {
            n121 = call "Timeout Selector.vi"("Remaining States"=w58, "Timeout Expected"=w61) -> ("Timeout"=w59:i32)  [unwired: 5 in]
            n122 = event shown="[0] Timeout" {
              selector: w60 -> [_ _ _]
              dyn-events: _ -> [_ _ _]
              timeout: w59 -> [_ _ _]
              tunnel: w58 -> [w70 w72 w79]
              tunnel: [w69 w72 w78] -> w66
              tunnel: w65 -> [w67 w73 w76]
              tunnel: [w68 w71 w77] -> w64
              tunnel: w63 -> [w68 w71 w77]
              tunnel: [w67 w73 w76] -> w62
              event Timeout {
                n123 = event-data() -> ()  [unwired: 1 in, 1 out]
                n124 = call <vilib>:"Add State(s) to Queue__JKI_lib_State_Machine.vi"("State(s) in (\"\")"=w70) -> ("States Out"=w69:string)  [unwired: 14 in]
              }
              event User Event {
                # "#CSM \"New State Notifier Event\"\nThis user event is used to break out CSM from waiting in the event structure, to process the next state from external. DO NOT place any code here unless you really need to."
                n125 = event-data() -> ()  [unwired: 1 in, 1 out]
              }
              event Panel Close? {
                # "#CSM Discard Panel Close?\nDiscard the event because we'll close the front panel ourselves in Macro: Exit"
                n126 = event-data() -> ()  [unwired: 1 in, 1 out]
                n127 = call <vilib>:"Add State(s) to Queue__JKI_lib_State_Machine.vi"("State(s) in Front (\"\")"="Macro: Exit", "State(s) in (\"\")"=w79) -> ("States Out"=w78:string)  [unwired: 13 in]
                n128 = event-data("Discard?"=TRUE) -> ()  [unwired: 1 in, 1 out]
              }
            }
          }
          frame "CSM Documentation" {
            # "#CSM README FIRST\n\nCommunicable State Machine(CSM) is a LabVIEW application framework that builds upon JKI State Machine(JKISM). It follows the pattern of JKISM and extends the keywords to describe message communication between modules, including concepts such as Sync-Message, Async-Message, Subscription/Unsubscription of status - essential elements for creating reusable code modules. For more information, please visit the CSM wiki: https://nevstop-lab.github.io/CSM-Wiki/\n\nFor instructions on JKI State Machine, visit: http://jki.net/state-machine/\nFor information about CSM, visit: https://github.com/NEVSTOP-LAB"
            # "#CSM \"Documentation\"\nCase for holding CSM Documenation"
          }
          frame "---------- Core ----------" {
            # "#CSM \"Category Seperator\"\nDo not put any code in this frame."
            n129 = call <vilib>:"Add State(s) to Queue__JKI_lib_State_Machine.vi"("State(s) in (\"\")"=w88) -> ("States Out"=w87:string)  [unwired: 14 in]
          }
          frame Default {
            # "#CSM \"Default\"\nthis is used to capture unhandled states and typos"
            # "Handle mistyped state name (developer tool)"
            n130 = call "CSM Unhandled State Error.vi"("error in (no error)"=w97, "Undefined State"=w91, "CSM Name"=w90) -> ("error out"=w89:errorcluster)  [unwired: 8 in]
            n131 = call <vilib>:"Add State(s) to Queue__JKI_lib_State_Machine.vi"("State(s) in (\"\")"=w96) -> ("States Out"=w95:string)  [unwired: 14 in]
          }
          frame "VI Reference" {
            n132 = Unbundle By Name(w102) -> ("Core"=w100:T4)
            n133 = Unbundle By Name(w100) -> ("Current VI Reference"=w99:refnum<vi>)
            n134 = call "CSM - Convert Data to HexStr.vi"("Variant"=w99) -> ("HEX String (0-9,A-F)"=w98:string)  [unwired: 8 in]
          }
          frame "Error Handler" {
            # "#CSM Disable this error dialog if you need"
            # "#CSM \"Error Handler\"\nYou can also output any states to clean-up after errors occur"
            # "Clear error"
            n135 = case shown="Error" w110 {
              selector: w110 -> [_ w120]
              tunnel: [w119 w122] -> w106
              tunnel: w109 -> [w119 w121]
              tunnel: w108 -> [w118 _]
              tunnel: [w117 w120] -> w111
              frame No Error {
                n136 = call "CSM - Convert Argument to Error.vi"("Argument"=w118) -> ("Error"=w117:errorcluster)  [unwired: 4 in]
                n137 = flat-sequence {
                  frame #0 {
                    # "#CSM External Error Handler Case\nUsually, it's because This CSM register others' \"Error Occurred\" status with \"Error Handler\". If other CSM have any error, the error will be passed here for central handling."
                  }
                }
              }
              frame Error {
                # "#CSM Internal Error Handler Case \nIf any error Occurred, \"Error Occurred\" \nstatus update will be broadcasted to system.\nParameter is Error Cluster."
                n138 = call "CSM - Convert Error to Argument.vi"("Error"=w120) -> ("Argument"=w124:string)  [unwired: 4 in]
                n139 = call <vilib>:"Build State String with Arguments__JKI_lib_State_Machine.vi"("Arguments (\"\")"=w124, "State"="Error Occurred" ("Status with Arguments")) -> ("State with Arguments"=w123:string)  [unwired: 4 in]
                n140 = call "CSM - Broadcast Status Change.vi"("Status With Arguments"=w123, "State Queue"=w121) -> ("Remaining States"=w122:string)  [unwired: 13 in]
              }
            }
            n141 = disable-structure shown="Enabled" {
              disable-tunnel: w111 -> [w115 w116]
              frame Enabled {
                n142 = call <vilib>:"General Error Handler.vi"("error in (no error)"=w115) -> ()  [unwired: 10 in, 5 out]
              }
              frame Disabled {
                n143 = call <vilib>:"Clear Errors.vi"("error in (no error)"=w116) -> ()  [unwired: 5 in, 2 out]
              }
            }
            n144 = call <vilib>:"Add State(s) to Queue__JKI_lib_State_Machine.vi"("State(s) in Front (\"\")"="// Post Error States", "State(s) in (\"\")"=w106) -> ("States Out"=w105:string)  [unwired: 13 in]
          }
          frame "Critical Error" {
            # "#CSM Stop in Critical Error\nWhen Critical Error occurs, Stop the loop immediately. Do NOT change this unless you fully understand the impact."
            # "#CSM \"Critical Error\"\nWhen any un-recoverable error occurs, CSM goes into this case."
            n145 = call "CSM Critical Error.vi"("error in (no error)"=w134, "Arugments (As Reason)"=w127, "CSM Name"=w126) -> ("error out"=w128:errorcluster)  [unwired: 8 in]
            n146 = call <vilib>:"Add State(s) to Queue__JKI_lib_State_Machine.vi"("State(s) in (\"\")"=w132) -> ("States Out"=w131:string)  [unwired: 14 in]
          }
          frame "Target Error" {
            # "#CSM \"Target Error\"\nWhen This CSM try to communicate with an un-existed CSM, This CSM goes into this case."
            n147 = call "CSM Target Error.vi"("error in (no error)"=w136, "Arguments (As CSM Name)"=w137) -> ("error out"=w135:errorcluster)  [unwired: 9 in]
            n148 = call <vilib>:"Add State(s) to Queue__JKI_lib_State_Machine.vi"("State(s) in (\"\")"=w138) -> ("States Out"=w141:string)  [unwired: 14 in]
          }
          frame "Target Timeout Error" {
            # "#CSM \"Target Timeout Error\"\nWhen This CSM could not get the sync-call response in time, This CSM goes into this case."
            n149 = call "CSM Target Timeout Error.vi"("error in (no error)"=w143, "Arguments (As CSM Name)"=w144) -> ("error out"=w142:errorcluster)  [unwired: 9 in]
            n150 = call <vilib>:"Add State(s) to Queue__JKI_lib_State_Machine.vi"("State(s) in (\"\")"=w145) -> ("States Out"=w148:string)  [unwired: 14 in]
          }
          frame "Async Response", "Response" {
            n151 = Unbundle(w154) -> ("’Error"=w150:errorcluster)  [unwired: 2 out]
            n152 = call <vilib>:"Add State(s) to Queue__JKI_lib_State_Machine.vi"("State(s) in (\"\")"=w151) -> ("States Out"=w152:string)  [unwired: 14 in]
            "Arguments" <- w149
          }
          frame "Async Message Posted" {
            # "#CSM \"Async Message Posted\"\nAfter Async Message is posted (-> or ->| ), CSM goes to this state for post-action.\nYou can use Argument - State to tell which Async Message is called."
          }
          frame "Initialize Core Data" {
            # "#CSM \"Initialize Core Data\"\nThis is used to determine panel behavior on exit"
            # "originally closed?"
            # "exe?"
            # "If panel starts closed or is an EXE, then close it when we exit"
            n153 = property class="VI"() -> ("FP.State"=w163:T1)  [unwired: 2 in, 2 out]
            n154 = property class="App"() -> ("App.Kind"=w169:T2)  [unwired: 2 in, 2 out]
            n155 = control-ref of="Current VI Reference"() -> (w164:refnum<vi>)
            n156 = Equal?(x=w163, y=T1."Closed" ("Front Panel Window:State")) -> (x = y?=w161:bool)
            n157 = Equal?(x=w169, y=T2."Run Time System" ("Application:Kind")) -> (x = y?=w167:bool)
            n158 = Or(x=w161, y=w167) -> (x .or. y?=w165:bool)
            n159 = Bundle By Name(cluster=w166, "Core.Current VI Reference"=w164, "Core.Close Panel on Exit?"=w165) -> (w171:T5)
            n160 = call <vilib>:"Add State(s) to Queue__JKI_lib_State_Machine.vi"("State(s) in (\"\")"=w173) -> ("States Out"=w172:string)  [unwired: 14 in]
          }
          frame "Exit" {
            # "#CSM \"Exit\"\nCase for exiting the loop. No errors that occur here will be handled."
            n161 = call <vilib>:"Add State(s) to Queue__JKI_lib_State_Machine.vi"("State(s) in (\"\")"=w179) -> ("States Out"=w178:string)  [unwired: 14 in]
          }
          frame "---------- Data ----------" {
            # "#CSM \"Category Seperator\"\nDo not put any code in this frame."
            n162 = call <vilib>:"Add State(s) to Queue__JKI_lib_State_Machine.vi"("State(s) in (\"\")"=w184) -> ("States Out"=w183:string)  [unwired: 14 in]
          }
          frame "Data: Initialize" {
            w186 = T4 {"Current VI Reference"=refnum, "Close Panel on Exit?"=FALSE}  # Core
            w188 = 0.0  # diff
            w187 = timestamp(0 s since 1904-01-01)  # time
            # "#CSM do not delete - used by framework"
            # "#CSM Expand Bundle to add new data elements to shift register data."
            # "Initialize the shift-register data, here.\n(data names are defined by what you wire into the bundle function)"
            n163 = Bundle("Core"=w186, "diff"=w188, "time"=w187) -> (w190:T5)  [unwired: 1 in]
            n164 = call <vilib>:"Add State(s) to Queue__JKI_lib_State_Machine.vi"("State(s) in (\"\")"=w192) -> ("States Out"=w191:string)  [unwired: 14 in]
          }
          frame "Data: Cleanup" {
            # "Cleanup any data and references, here.\n(this is called automatically, by the Macro: Exit)"
            n165 = Unbundle By Name(w194) -> ("Core.Current VI Reference"=w197:refnum<vi>)
            n166 = Close Reference(reference=w197, error in (no error)=w196) -> (error out=w195:errorcluster)
            n167 = call <vilib>:"Add State(s) to Queue__JKI_lib_State_Machine.vi"("State(s) in (\"\")"=w199) -> ("States Out"=w198:string)  [unwired: 14 in]
          }
          frame "---------- Events ----------" {
            # "#CSM \"Category Seperator\"\nDo not put any code in this frame."
            n168 = call <vilib>:"Add State(s) to Queue__JKI_lib_State_Machine.vi"("State(s) in (\"\")"=w204) -> ("States Out"=w203:string)  [unwired: 14 in]
          }
          frame "Events: Register" {
            # "#CSM \"Events: Register\"\nRegister user event. New Message Event is registered to break CSM waiting in event structure by default."
            # "#CSM Register New Message Event\nRegister message event to break Waiting in Event structure."
            n169 = call "CSM - Get New State Notifier Event.vi"("Name (\"\" to Use UUID)"=w208) -> ("error out"=w206:errorcluster, "New State Notifier Event"=w207:refnum<user-event>)  [unwired: 9 in]
            n170 = register-events(error in=w206, w207) -> (reference out=w209:refnum<event-registration>, error out=w205:errorcluster)  [unwired: 1 in]
          }
          frame "Events: Unregister" {
            # "#CSM \"Events: Unregister\"\nUnregister user event."
            n171 = Unregister For Events(event registration refnum=w212, error in=w216) -> (error out=w213:errorcluster)
          }
          frame "---------- UI ----------" {
            # "#CSM \"Category Seperator\"\nDo not put any code in this frame."
            n172 = call <vilib>:"Add State(s) to Queue__JKI_lib_State_Machine.vi"("State(s) in (\"\")"=w221) -> ("States Out"=w220:string)  [unwired: 14 in]
          }
          frame "UI: Initialize" {
            # "#CSM \"UI: Initialize\"\nInitialize the User Interface, here.\n(this is called automatically, by the Macro: Init)"
            n173 = call <vilib>:"Add State(s) to Queue__JKI_lib_State_Machine.vi"("State(s) in (\"\")"=w227) -> ("States Out"=w226:string)  [unwired: 14 in]
            n174 = local write "Arguments"("" ("Arguments")) -> ()
          }
          frame "UI: Cursor Set" {
            # "#CSM \"UI: Cursor Set\"\nSet and Unset Cursor Busy.\n(Usage: \"UI: Cursor Set >> Busy|Idle\")"
            # "Argument"
            n175 = disable-structure shown="Default" {
              disable-tunnel: w231 -> [w237 w242]
              disable-tunnel: [w236 w242] -> w230
              disable-tunnel: w229 -> [w235 _]
              frame condition #0 (active) {
                n176 = case shown="\"Idle\", Default" w235 {
                  tunnel: w237 -> [w239 w241]
                  tunnel: [w238 w240] -> w236
                  frame "Idle", Default {
                    n177 = call <vilib>:"Unset Busy.vi"("error in (no error)"=w239) -> ("error out"=w238:errorcluster)  [unwired: 10 in]
                  }
                  frame "Busy" {
                    n178 = call <vilib>:"Set Busy.vi"("error in (no error)"=w241) -> ("error out"=w240:errorcluster)  [unwired: 9 in, 1 out]
                  }
                }
              }
              frame condition #1 {
              }
            }
            n179 = call <vilib>:"Add State(s) to Queue__JKI_lib_State_Machine.vi"("State(s) in (\"\")"=w234) -> ("States Out"=w233:string)  [unwired: 14 in]
          }
          frame "UI: Front Panel State" {
            # "#CSM \"UI: Front Panel State\"\nSet Front Panel Open or Closed\n(Usage: \"UI: Front Panel State >> Open|Close\")"
            # "Argument"
            n180 = Unbundle By Name(w246) -> ("Core.Current VI Reference"=w245:refnum<vi>)
            n181 = call <vilib>:"Add State(s) to Queue__JKI_lib_State_Machine.vi"("State(s) in (\"\")"=w250) -> ("States Out"=w249:string)  [unwired: 14 in]
            n182 = case shown="\"Close\", \"Closed\"" w244 {
              tunnel: w248 -> [w256 w271 w282 w295 w308]
              tunnel: [w258 w272 w284 w297 w310] -> w247
              tunnel: w245 -> [w257 w269 w283 w296 w309]
              frame "Open", "Standard", Default {
                w251 = T1."Standard" ("State")
                n183 = property class="VI"(reference=w257, error in=w256) -> (reference out=w254:refnum<vi>, error out=w255:errorcluster, "FP.State"=w253:T1)
                n184 = Not Equal?(x=w253, y=w251) -> (x != y?=w252:bool)
                n185 = case shown="True" w252 {
                  tunnel: [w262 w264] -> w258
                  tunnel: w255 -> [w261 w264]
                  tunnel: w254 -> [w260 _]
                  tunnel: w251 -> [w259 _]
                  frame True {
                    n186 = invoke class="VI" method="FP.Open"(reference=w260, error in=w261, "Activate"=TRUE, "State"=w259) -> (error out=w262:errorcluster)  [unwired: 1 in, 4 out]
                  }
                  frame False {
                  }
                }
              }
              frame "Close", "Closed" {
                n187 = property class="VI"(reference=w269, error in=w271) -> (reference out=w268:refnum<vi>, error out=w270:errorcluster, "FP.State"=w266:T1)
                n188 = Not Equal?(x=w266, y=T1."Closed" ("Front Panel Window:State")) -> (x != y?=w265:bool)
                n189 = case shown="False" w265 {
                  tunnel: [w273 w276] -> w272
                  tunnel: w270 -> [w273 w275]
                  tunnel: w268 -> [_ w274]
                  frame False {
                  }
                  frame True {
                    n190 = invoke class="VI" method="FP.Close"(reference=w274, error in=w275) -> (error out=w276:errorcluster)  [unwired: 1 in, 2 out]
                  }
                }
              }
              frame "Hidden", "Hide" {
                w277 = T1."Hidden" ("State")
                n191 = property class="VI"(reference=w283, error in=w282) -> (reference out=w280:refnum<vi>, error out=w281:errorcluster, "FP.State"=w279:T1)
                n192 = Not Equal?(x=w279, y=w277) -> (x != y?=w278:bool)
                n193 = case shown="True" w278 {
                  tunnel: [w288 w289] -> w284
                  tunnel: w281 -> [w287 w289]
                  tunnel: w280 -> [w286 _]
                  tunnel: w277 -> [w285 _]
                  frame True {
                    n194 = invoke class="VI" method="FP.Open"(reference=w286, error in=w287, "State"=w285) -> (error out=w288:errorcluster)  [unwired: 2 in, 4 out]
                  }
                  frame False {
                  }
                }
              }
              frame "Minimize", "Minimized" {
                w290 = T1."Minimized" ("State")
                n195 = property class="VI"(reference=w296, error in=w295) -> (reference out=w293:refnum<vi>, error out=w294:errorcluster, "FP.State"=w292:T1)
                n196 = Not Equal?(x=w292, y=w290) -> (x != y?=w291:bool)
                n197 = case shown="True" w291 {
                  tunnel: [w301 w302] -> w297
                  tunnel: w294 -> [w300 w302]
                  tunnel: w293 -> [w299 _]
                  tunnel: w290 -> [w298 _]
                  frame True {
                    n198 = invoke class="VI" method="FP.Open"(reference=w299, error in=w300, "State"=w298) -> (error out=w301:errorcluster)  [unwired: 2 in, 4 out]
                  }
                  frame False {
                  }
                }
              }
              frame "Maximize", "Maximized" {
                w303 = T1."Maximized" ("State")
                n199 = property class="VI"(reference=w309, error in=w308) -> (reference out=w306:refnum<vi>, error out=w307:errorcluster, "FP.State"=w305:T1)
                n200 = Not Equal?(x=w305, y=w303) -> (x != y?=w304:bool)
                n201 = case shown="True" w304 {
                  tunnel: [w314 w315] -> w310
                  tunnel: w307 -> [w313 w315]
                  tunnel: w306 -> [w312 _]
                  tunnel: w303 -> [w311 _]
                  frame True {
                    n202 = invoke class="VI" method="FP.Open"(reference=w312, error in=w313, "State"=w311) -> (error out=w314:errorcluster)  [unwired: 2 in, 4 out]
                  }
                  frame False {
                  }
                }
              }
            }
          }
          frame "---------- Macro ----------" {
            # "#CSM \"Category Seperator\"\nDo not put any code in this frame."
            n203 = call <vilib>:"Add State(s) to Queue__JKI_lib_State_Machine.vi"("State(s) in (\"\")"=w320) -> ("States Out"=w319:string)  [unwired: 14 in]
          }
          frame "Macro: Initialize" {
            w322 = "Data: Initialize\nInitialize Core Data\nEvents: Register\nUI: Initialize\nUI: Front Panel State >> Open"  # Data: Initialize Initialize Core Data Events: Register UI: Initialize UI: Front Panel State >> Open
            # "#CSM \"Macro: Initialize\"\nInitialization Macro (This is called once, when the VI starts)"
            n204 = call <vilib>:"Add State(s) to Queue__JKI_lib_State_Machine.vi"("State(s) in Front (\"\")"=w322, "State(s) in (\"\")"=w326) -> ("States Out"=w325:string)  [unwired: 13 in]
          }
          frame "Macro: Exit" {
            # "#CSM \"Macro: Exit\"\nExit Macro (This is called once, when the VI exits)"
            n205 = Unbundle By Name(w335) -> ("Core.Close Panel on Exit?"=w334:bool)
            n206 = Select(t="UI: Front Panel State >> Close", s=w334, f="") -> (s? t:f=w331:string)
            n207 = call <vilib>:"Add State(s) to Queue__JKI_lib_State_Machine.vi"("State(s) in Front (\"\")"="//Exit Sub-Modules ", "State(s) in (\"\")"=w331, "State(s) at Back (\"\")"="Data: Cleanup\nEvents: Unregister\nExit") -> ("States Out"=w329:string)  [unwired: 12 in]
            n208 = call <vilib>:"Add State(s) to Queue__JKI_lib_State_Machine.vi"("State(s) in Front (\"\")"=w329, "State(s) in (\"\")"=w338) -> ("States Out"=w337:string)  [unwired: 13 in]
          }
          frame "---------- API ----------" {
            # "#CSM \"Category Seperator\"\nDo not put any code in this frame."
          }
          frame "API: API1" {
            # "#CSM API Example\nCopy/Rename this case for your own API"
            # "#CSM Response\nConnect this to return the response of your API"
            # "#CSM >> Source CSM >>\nIf you need to tell who triggered this state , use this string. If it's this case itself, this string is \"\"."
            # "#CSM >> Arguments >>\nDeal with the parameter if any"
          }
          frame "API: API2" {
            # "#CSM API Example\nCopy/Rename this case for your own API"
            # "unpack Hex String  to Variant\nif complex parameter is needed."
            n209 = call "CSM - Convert HexStr to Data.vi"("HEX String"=w349) -> ()  [unwired: 7 in, 2 out]
            n210 = disable-structure shown="Disabled" {
              disable-tunnel: [w354 "API2 Response"] -> w348
              frame Disabled {
                # "pack variant to hexstr \nif complex response is needed."
                # "complex Response"
                n211 = call "CSM - Convert Data to HexStr.vi"() -> ("HEX String (0-9,A-F)"=w354:string)  [unwired: 9 in]
              }
              frame Enabled {
              }
            }
          }
        }
      }
      n212 = call "CSM - Send Message and Wait for Reply.vi"("Response Timeout (-2 Using Global Settings)"=w5, "Error In (No Error)"=w21, "Target Module"=w11, "State"=w8) -> ("error out"=w10:errorcluster)  [unwired: 5 in, 2 out]
      n213 = call "CSM - Send Message and Wait for Reply.vi"("Response Timeout (-2 Using Global Settings)"=w5, "Error In (No Error)"=w10, "Target Module"="caller" ("Name (\"\" to Use UUID)"), "State"=w8) -> ("error out"=w9:errorcluster)  [unwired: 5 in, 2 out]
      n214 = flat-sequence {
        tunnel: w24 -> [w37]
        tunnel: [w36] -> w23
        tunnel: [w35] -> w22
        tunnel: w9 -> [w33]
        frame #0 {
          n215 = local read "Arguments"() -> (w32:string)
          n216 = call-dynamic "passIfEqual.vi"("error in (no error)"=w33, "y"="Done" ("HEX String (0-9,A-F)"), "x"=w32, "TestCase in"=w37) -> ("error out"=w35:errorcluster, "TestCase out"=w36:refnum<class "testcase-csm loop support.lvclass">)  [unwired: 6 in]
        }
      }
    }
    frame Disabled {
      # "skip test result while test is under development"
      n217 = call <vilib>:"skip.vi"("error in (no error)"=w724, "TestCase in"=w727) -> ("error out"=w726:errorcluster, "TestCase out"=w725:refnum<class "testcase-csm loop support.lvclass">)  [unwired: 8 in]
    }
  }
  "error out" <- w3
  "TestCase out" <- w1
